vi "Add New Option.vi"(8 "error in (no error)":errorcluster, 9 "Sort (T)":bool=TRUE, 10 "New Option":string, 11 "Shared Options in":refnum<class "Shared Options.lvclass">) -> (0 "error out":errorcluster, 3 "Shared Options out":refnum<class "Shared Options.lvclass">)   [LabVIEW 2020, in "AutoComplete.lvlib" / "Shared Options.lvclass"]
doc: "Adds a new option if it doesn't already exist so it is safe to call this VI for items that were selected from the available list. By default will re-sort options after adding a new element but that can be turned off."
uses:
  Shared Options.lvclass
  Shared Options.lvclass/Shared Options.ctl
  f4f2d3f9-33bc-4369-8649-e7d8ec0826f4.vi
  <vilib>/Comparison/Less/Less Functor/Less Functor.lvclass
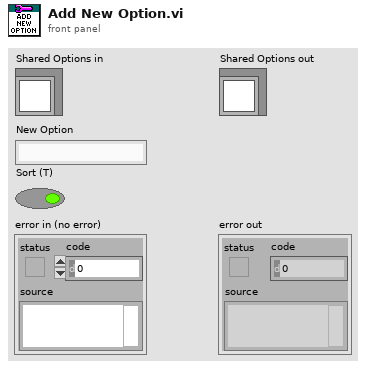
[diagram p1: front panel]
types:
  T1 = typedef "AutoComplete.lvlib/Options.ctl" = cluster{"Options":string[], "Allow Undefined Values":bool}
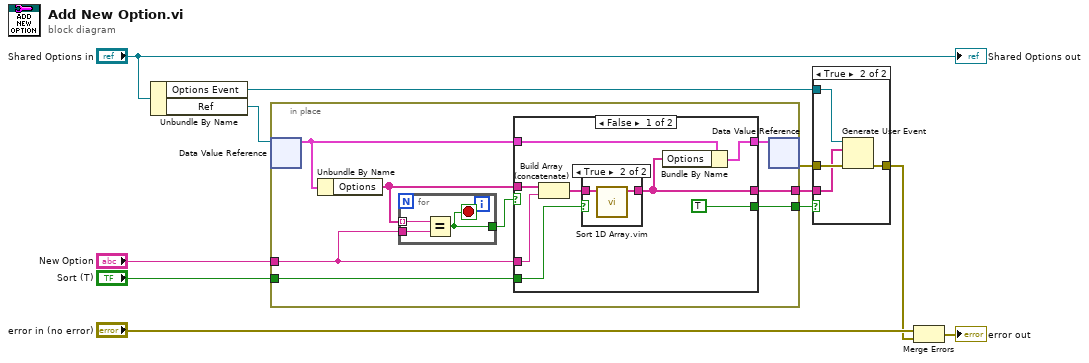
[diagram p0: block diagram]
diagram:
  n1 = Unbundle By Name("Shared Options in") -> ("Options Event"=w3:refnum<user-event>, "Ref"=w9:refnum<data-value>)
  n2 = in-place {
    in-place-border: "New Option" -> [w15]
    in-place-border: "Sort (T)" -> [w14]
    in-place-border: [w13] -> w5
    in-place-border: [w12] -> w4
    n3 = in-place-dvr #1(w9) -> (w17:T1)  [unwired: 1 out]
    n4 = Unbundle By Name(w17) -> ("Options"=w18:string[])
    n5 = for {
      tunnel: w15 -> [w33]
      tunnel: w18 -> [w34] mode=indexing
      tunnel: [w32] -> w19
      stop <- w32 stop-if-true
      n6 = Equal?(x=w34, y=w33) -> (x = y?=w32:bool)
    }
    n7 = case shown="False" w19 {
      tunnel: w18 -> [w27 _]
      tunnel: w17 -> [w22 w31]
      tunnel: [w23 w31] -> w16
      tunnel: w15 -> [w26 _]
      tunnel: w14 -> [w25 _]
      tunnel: [w21 _] -> w13
      tunnel: [TRUE _] -> w12
      frame False {
        n8 = Build Array (concatenate)(w27, w26) -> (w24:string[])
        n9 = case shown="True" w25 {
          tunnel: w24 -> [w28 w30]
          tunnel: [w28 w29] -> w21
          frame False {
          }
          frame True {
            n10 = call "Sort 1D Array.vim"("unsorted array"=w30) -> ("sorted array"=w29:string[])  [unwired: 10 in]
          }
        }
        n11 = Bundle By Name(cluster=w22, "Options"=w21) -> (w23:T1)
      }
      frame True {
      }
    }
    n12 = in-place-dvr #1(w16) -> (w7:errorcluster)  [unwired: 1 out]
  }
  n13 = case shown="True" w4 {
    tunnel: w7 -> [w35 w38]
    tunnel: w5 -> [_ w37]
    tunnel: w3 -> [_ w39]
    tunnel: [w35 w36] -> w1
    frame False {
    }
    frame True {
      n14 = Generate User Event(user event=w39, event data cluster=w37, error in=w38) -> (error out=w36:errorcluster)  [unwired: 1 in, 1 out]
    }
  }
  n15 = Merge Errors("error in (no error)", w1) -> (→"error out":errorcluster)
  "Shared Options out" <- "Shared Options in"
